vi "U64-to-U8Array.vi"(11 "Numeric":u64 format="%.0x") -> (3 "Array":u8[](array[numeric]) format="%.0x")   [LabVIEW 2017]
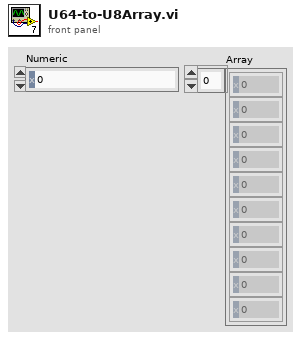
[diagram p1: front panel]
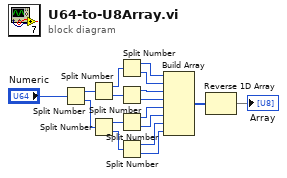
[diagram p0: block diagram]
diagram:
  n1 = Split Number(x="Numeric") -> (hi(x)=w4:u32, lo(x)=w5:u32)
  n2 = Split Number(x=w4) -> (hi(x)=w6:u16, lo(x)=w7:u16)
  n3 = Split Number(x=w5) -> (hi(x)=w8:u16, lo(x)=w9:u16)
  n4 = Split Number(x=w6) -> (hi(x)=w10:u8, lo(x)=w11:u8)
  n5 = Split Number(x=w7) -> (hi(x)=w12:u8, lo(x)=w13:u8)
  n6 = Split Number(x=w8) -> (hi(x)=w14:u8, lo(x)=w15:u8)
  n7 = Split Number(x=w9) -> (hi(x)=w17:u8, lo(x)=w16:u8)
  n8 = Build Array(w10, w11, w12, w13, w14, w15, w17, w16) -> (w2:u8[])
  n9 = Reverse 1D Array(array=w2) -> (reversed array=→"Array":u8[])
